vi "ReadTree.vi"(8 "error in":errorcluster, 10 "root":T1, 11 "CEF_Hierachy repository in":refnum<class "CEF_HierarchyRepo.lvclass">) -> (0 "error out":errorcluster, 3 "CEF_Hierachy repository out":refnum<class "CEF_Repository.lvclass">)   [LabVIEW 2025, in "CEF.lvlib" / "CEF_HierarchyRepo.lvclass"]
doc: "Transfers information between the repo and the tree control nodes. This should be called before custom views are launched or saving to disk.Copyright 2017 National Instruments Corporation\n\nLicensed under the Apache License, Version 2.0 (the \"License\"); you may not use this file except in compliance with the License. You may obtain a copy of the License at http://www.apache.org/licenses/LICENSE-2.0\nUnless required by applicable law or agreed to in writing, software distributed under the License is distributed on an \"AS IS\" BASIS, WITHOUT WARRANTIES OR CONDITIONS OF ANY KIND, either express or implied. See the License for the specific language governing permissions and limitations under the License."
uses:
  CEF_HierarchyRepo.lvclass
  Repository/CEF_Repository.lvclass
  Node/NodeRef.ctl
  Node/CEF_Node.lvclass
  memory hierarchy.ctl
  full hierarchy.ctl
  tree serializer/hierarchy element.ctl
  serializable configuration/CEF_serializable configuration.lvclass
  CEF_HierarchyRepo.lvclass/CEF_HierarchyRepo.ctl
  CEF.lvlib
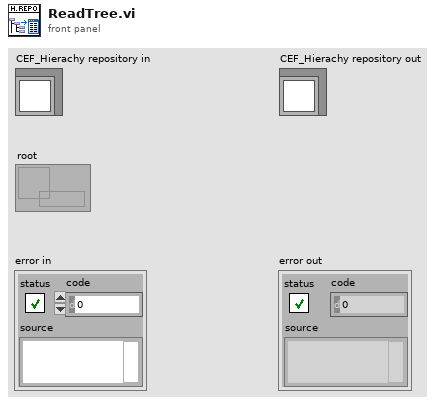
[diagram p1: front panel]
types:
  T1 = typedef "CEF.lvlib/CEF_Node.lvclass/NodeRef.ctl" = refnum<data-value>
  T2 = typedef "CEF.lvlib/CEF_HierarchyRepo.lvclass/memory hierarchy.ctl" = cluster{"hierarchy structure":T3, "instance data":refnum<class "CEF_serializable configuration.lvclass">[]}
  T3 = typedef "CEF.lvlib/CEF_HierarchyRepo.lvclass/full hierarchy.ctl" = cluster{"root":string, "hierarchy":T4[]}
  T4 = typedef "CEF.lvlib/hierarchy element.ctl" = cluster{"current node":string, "children":string[]}
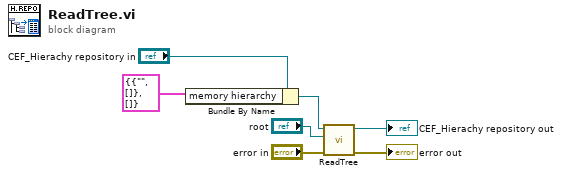
[diagram p0: block diagram]
diagram:
  n1 = Bundle By Name(cluster="CEF_Hierachy repository in", "memory hierarchy"=T2 {"hierarchy structure"={"root"="", "hierarchy"=[]}, "instance data"=[]}) -> (w3:refnum<class "CEF_HierarchyRepo.lvclass">)
  n2 = call-parent "ReadTree.vi"("error in"="error in", "root"="root", "CEF_Repository in"=w3) -> ("error out"=→"error out":errorcluster, "CEF_Repository out"=→"CEF_Hierachy repository out":refnum<class "CEF_Repository.lvclass">)  [unwired: 7 in]
